vi "Debug Flags.vi"(11 "Sequence Config in":refnum<class "Sequence Config.lvclass">) -> (2 "Debug":T1, 3 "Sequence Config out":refnum<class "Sequence Config.lvclass">)   [LabVIEW 2023, in "VolatusSeqConfig.lvlib" / "Sequence Config.lvclass"]
uses:
  Sequence Config.lvclass
  Sequence Config.lvclass/Sequence Config.ctl
  Debug Flags.ctl
  VolatusSeqConfig.lvlib
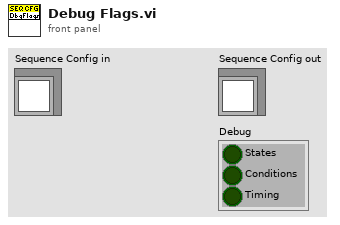
[diagram p1: front panel]
types:
  T1 = typedef "VolatusSeqConfig.lvlib/Debug Flags.ctl" = cluster{"States":bool, "Conditions":bool, "Timing":bool}
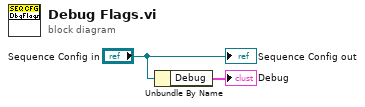
[diagram p0: block diagram]
diagram:
  n1 = Unbundle By Name("Sequence Config in") -> ("Debug"=→"Debug":T1)
  "Sequence Config out" <- "Sequence Config in"
